vi "Make Message.vi"(8 "error in (no error)":errorcluster, 9 "Message Type":T1, 10 "Method Qualified Name":string, 11 "Message Maker in":refnum<class "Message Maker.lvclass">) -> (0 "error out":errorcluster, 3 "Message Maker out":refnum<class "Message Maker.lvclass">)   [LabVIEW 2023, in "Message Maker.lvclass"]
doc: "Builds a message for the method specified\n\nAuthor: Derek Trepanier\nCopyright: MGI 2015"
uses:
  Message Maker.lvclass
  Message Maker.lvclass/Message Maker.ctl
  Message Status.ctl
  Message Type.ctl
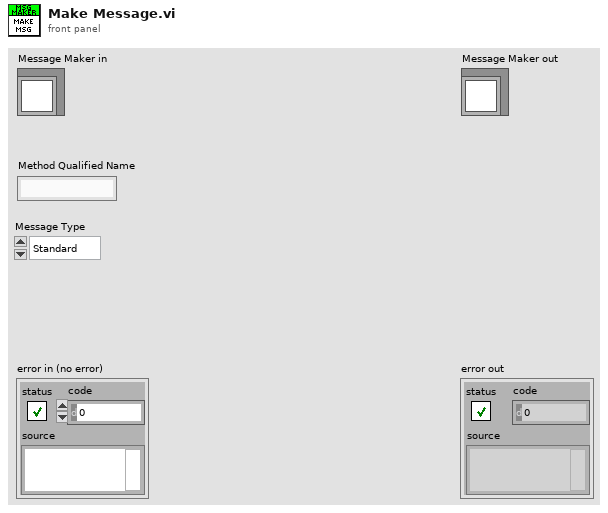
[diagram p1: front panel]
types:
  T1 = typedef "Message Maker.lvclass/Message Type.ctl" = enum16{"Standard", "Async"}
  T2 = typedef "Message Maker.lvclass/Message Status.ctl" = enum16{"Message Not Created", "Message Out of Date", "Message OK", "Never update"}
  T3 = typedef "Message Maker.lvclass/Scripting Refs.ctl" = cluster{"Actor Method VI":refnum<vi>, "Actor Class":refnum<vi>, "Message Class":refnum<vi>}
  T4 = typedef "Message Maker.lvclass/Message Recipient Type.ctl" = enum16{"Actor", "Interface"}
  T5 = typedef "Message Maker.lvclass/Wiring Spec.ctl" = cluster{"Actor":cluster{"In":i32, "Out":i32}, "Error":cluster{"In":i32, "Out":i32}, "Terminals":cluster{"Position":T6, "Terminal":i32}[]}
  T6 = typedef "Message Maker.lvclass/Connector Pane Position.ctl" = enum16{"Left", "Top", "Bottom", "Right"}
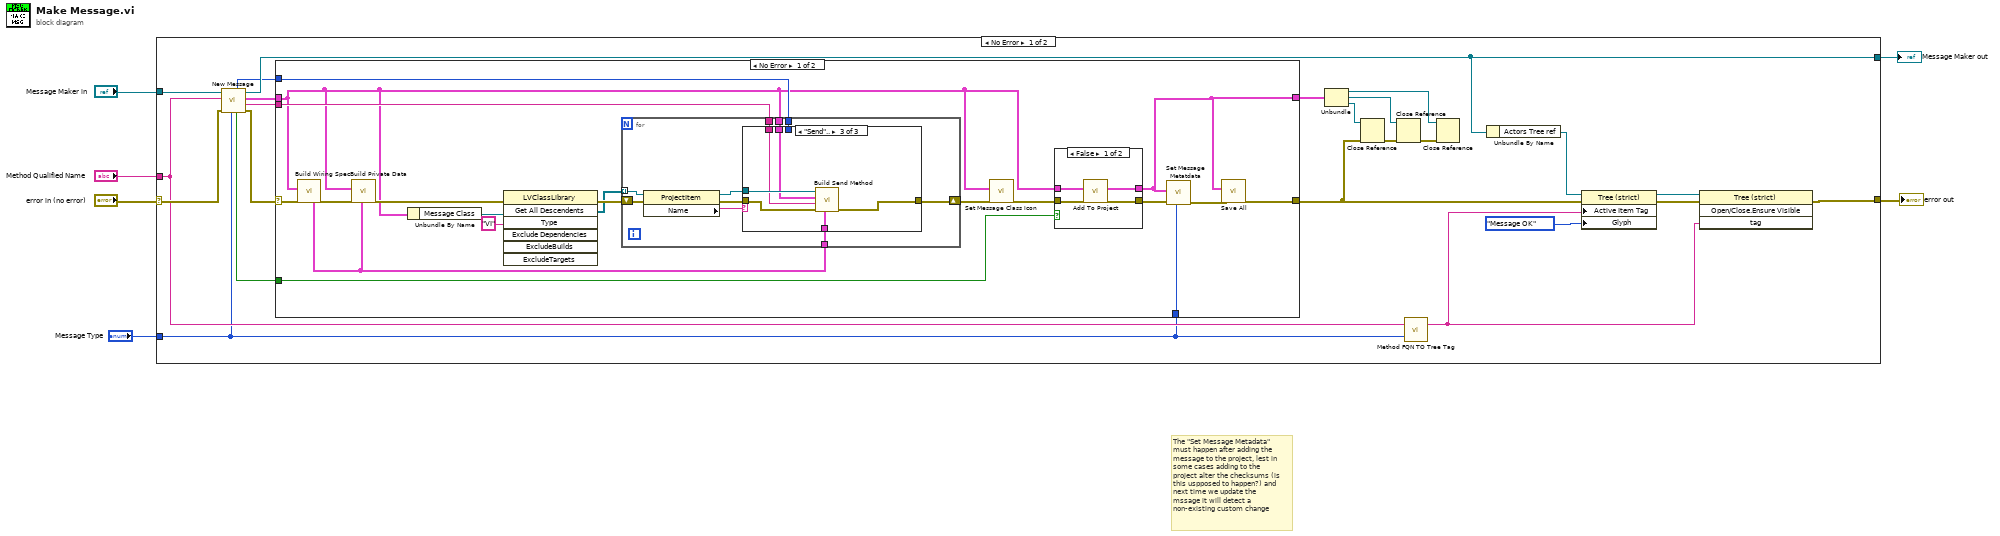
[diagram p0: block diagram]
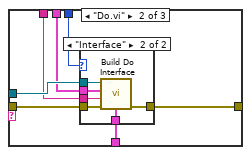
[diagram p4: hidden frame]
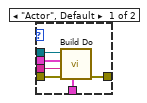
[diagram p5: hidden frame]
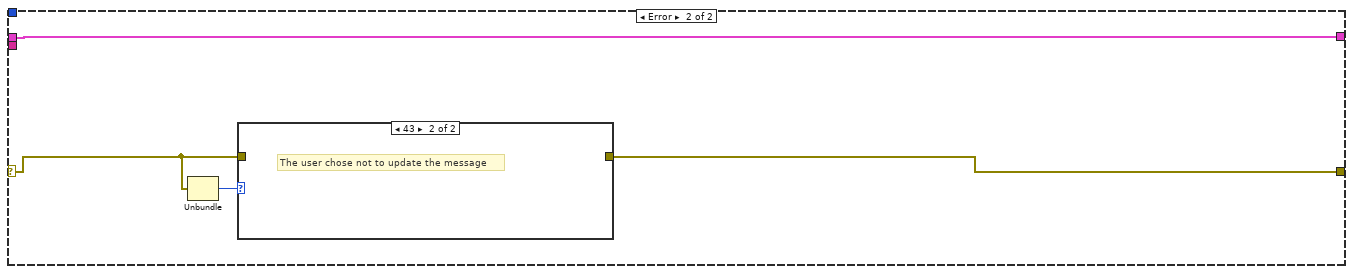
[diagram p6: hidden frame]
diagram:
  # "The \"Set Message Metadata\" must happen after adding the message to the project, lest in some cases adding to the project alter the checksums (is this uspposed to happen?) and next time we update the mssage it will detect a non-existing custom change"
  n1 = case shown="No Error" "error in (no error)" {
    selector: "error in (no error)" -> [w29 w97]
    tunnel: [w12 w97] -> w5
    tunnel: [w18 w96] -> w3
    tunnel: "Message Maker in" -> [w28 w96]
    tunnel: "Method Qualified Name" -> [w9 _]
    tunnel: "Message Type" -> [w7 _]
    frame No Error {
      n2 = call "New Message.vi"("Message Type"=w7, "error in (no error)"=w29, "Method Qualified Name"=w9, "Message Maker in"=w28) -> ("error out"=w19:errorcluster, "AF Library FQN"=w11:string, "References"=w23:T3, "Message Maker out"=w18:refnum<class "Message Maker.lvclass">, "Updating?"=w24:bool, "Message Recipient Type"=w10:T4)  [unwired: 2 in]
      n3 = case shown="No Error" w19 {
        selector: w19 -> [w38 w92]
        tunnel: w24 -> [w41 _]
        tunnel: w23 -> [w32 w94]
        tunnel: [w40 w91] -> w16
        tunnel: [w31 w94] -> w20
        tunnel: w11 -> [w37 _]
        tunnel: w10 -> [w36 _]
        tunnel: w7 -> [w30 _]
        frame No Error {
          n4 = call "Build Wiring Spec.vi"("error in (no error)"=w38, "References"=w32) -> ("error out"=w48:errorcluster, "Wiring Spec"=w43:T5)  [unwired: 8 in]
          n5 = call "Build Private Data.vi"("Wiring Spec"=w43, "error in (no error)"=w48, "References"=w32) -> ("error out"=w44:errorcluster)  [unwired: 8 in]
          n6 = Unbundle By Name(w32) -> ("Message Class"=w42:refnum<vi>)
          n7 = invoke class="LVClassLibrary" method="Get All Descendents"(reference=w42, error in=w44, "Type"="VI") -> (error out=w47:errorcluster, "All Descendents"=w46:refnum<vi>[])  [unwired: 4 in, 5 out]
          n8 = for {
            tunnel: w46 -> [w64] mode=indexing
            shift-right: [w59] -> w39
            shift-left: w47 -> [w61]
            tunnel: w32 -> [w58]
            tunnel: w43 -> [w57]
            tunnel: w37 -> [w56]
            tunnel: w36 -> [w55]
            n9 = property class="ProjectItem"(reference=w64, error in=w61) -> (reference out=w62:refnum<vi>, error out=w60:errorcluster, "Name"=w63:string)
            n10 = case shown="\"Send\".." w63 {
              tunnel: w62 -> [_ w72 w90]
              tunnel: w60 -> [w65 w71 w88]
              tunnel: [w65 w70 w89] -> w59
              tunnel: w58 -> [_ w68 w87]
              tunnel: w57 -> [_ w69 w86]
              tunnel: w56 -> [_ w67 w85]
              tunnel: w55 -> [_ w66 _]
              frame Default {
              }
              frame "Do.vi" {
                n11 = case shown="\"Interface\"" w66 {
                  tunnel: w72 -> [w78 w82]
                  tunnel: w71 -> [w77 w84]
                  tunnel: [w76 w83] -> w70
                  tunnel: w69 -> [w75 w79]
                  tunnel: w68 -> [w74 w81]
                  tunnel: w67 -> [w73 w80]
                  frame "Actor", Default {
                    n12 = call "Build Do.vi"("Wiring Spec"=w75, "error in (no error)"=w77, "AF Library FQN"=w73, "References"=w74, "Do VI"=w78) -> ("error out"=w76:errorcluster)  [unwired: 6 in]
                  }
                  frame "Interface" {
                    n13 = call "Build Do Interface.vi"("Wiring Spec"=w79, "error in (no error)"=w84, "AF Library FQN"=w80, "References"=w81, "Do VI"=w82) -> ("error out"=w83:errorcluster)  [unwired: 6 in]
                  }
                }
              }
              frame "Send".. {
                n14 = call "Build Send Method.vi"("Wiring Spec"=w86, "error in (no error)"=w88, "AF Library FQN"=w85, "References"=w87, "Send VI"=w90) -> ("error out"=w89:errorcluster)  [unwired: 6 in]
              }
            }
          }
          n15 = call "Set Message Class Icon.vi"("error in (no error)"=w39, "References"=w32) -> ("error out"=w35:errorcluster)  [unwired: 9 in]
          n16 = case shown="False" w41 {
            tunnel: w35 -> [w52 w54]
            tunnel: w32 -> [w51 w53]
            tunnel: [w50 w54] -> w34
            tunnel: [w49 w53] -> w31
            frame False {
              n17 = call "Add To Project.vi"("error in (no error)"=w52, "References"=w51) -> ("error out"=w50:errorcluster, "Out"=w49:T3)  [unwired: 8 in]
            }
            frame True {
            }
          }
          n18 = call "Set Message Metatdata.vi"("Message Type"=w30, "error in (no error)"=w34, "References"=w31) -> ("error out"=w33:errorcluster)  [unwired: 8 in]
          n19 = call "Save All.vi"("error in (no error)"=w33, "References"=w31) -> ("error out"=w40:errorcluster)  [unwired: 9 in]
        }
        frame Error {
          n20 = Unbundle(w92) -> ("code"=w93:i32)  [unwired: 2 out]
          n21 = case shown="43" w93 {
            tunnel: w92 -> [w95 _]
            tunnel: [w95 _] -> w91
            frame 0, Default {
            }
            frame 43 {
              # "The user chose not to update the message"
            }
          }
        }
      }
      n22 = Unbundle(w20) -> ("Actor Method VI"=w27:refnum<vi>, "Actor Class"=w26:refnum<vi>, "Message Class"=w25:refnum<vi>)
      n23 = Close Reference(reference=w25, error in (no error)=w16) -> (error out=w21:errorcluster)
      n24 = Close Reference(reference=w26, error in (no error)=w21) -> (error out=w22:errorcluster)
      n25 = call "Method FQN TO Tree Tag.vi"("Message Type"=w7, "Method FQN"=w9) -> ("Method Tree Tag"=w8:string)  [unwired: 1 in]
      n26 = Close Reference(reference=w27, error in (no error)=w22) -> ()  [unwired: 1 out]
      n27 = Unbundle By Name(w18) -> ("Actors Tree ref"=w17:refnum<vi>)
      n28 = property class="Tree (strict)"(reference=w17, error in=w16, "Active Item Tag"=w8, "Glyph"=Message_Status."Message OK" ("Message Status")) -> (reference out=w14:refnum<vi>, error out=w13:errorcluster)
      n29 = invoke class="Tree (strict)" method="Open/Close.Ensure Visible"(reference=w14, error in=w13, "tag"=w8) -> (error out=w12:errorcluster)  [unwired: 1 in, 3 out]
    }
    frame Error {
    }
  }
  "error out" <- w5
  "Message Maker out" <- w3
